vi "Practica 6 Alejandro Tejada ITIW31.vi"() -> ()   [LabVIEW 2018]
panel:
  in  "Eficiencia %":dbl
  out "Ganandia (dB)":dbl
  out "Longitud de onda":dbl
  in  "Frecuencia GHz (f)":dbl
  out "Area":dbl
  in  "Radio de la antena (r)":dbl
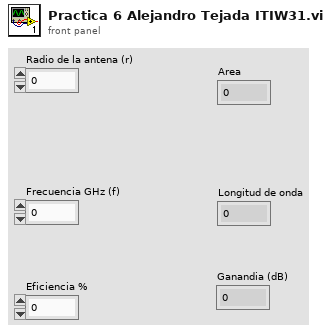
[diagram p1: front panel]
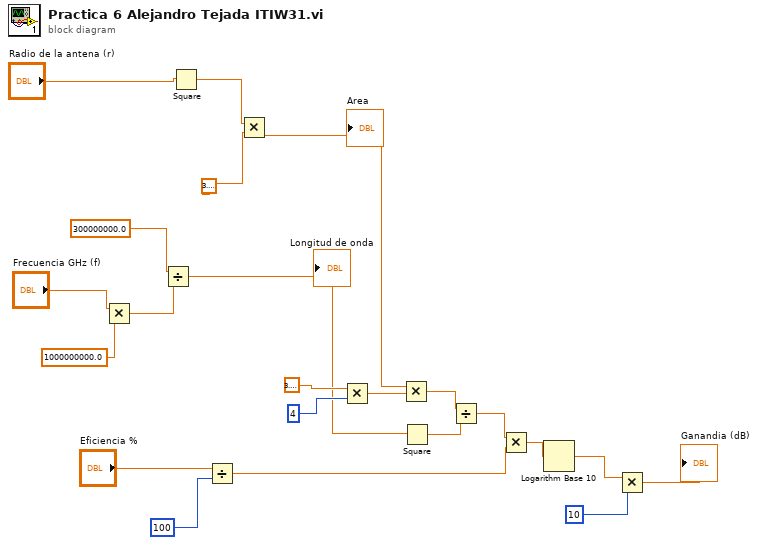
[diagram p0: block diagram]
diagram:
  n1 = Multiply(x="Frecuencia GHz (f)", y=1000000000.0) -> (x*y=w16:dbl)
  n2 = Divide(x=300000000.0, y=w16) -> (x/y=w9:dbl)
  "Longitud de onda" <- w9
  n3 = Square(x="Radio de la antena (r)") -> (x^2=w21:dbl)
  n4 = Divide(x="Eficiencia %", y=100) -> (x/y=w6:dbl)
  n5 = Multiply(x=w21, y=3.141592653589793) -> (x*y=w11:dbl)
  "Area" <- w11
  n6 = Multiply(x=3.141592653589793, y=4) -> (x*y=w10:dbl)
  n7 = Multiply(x=w11, y=w10) -> (x*y=w8:dbl)
  n8 = Square(x=w9) -> (x^2=w7:dbl)
  n9 = Divide(x=w8, y=w7) -> (x/y=w5:dbl)
  n10 = Multiply(x=w5, y=w6) -> (x*y=w2:dbl)
  n11 = Logarithm Base 10(1:w2) -> (0:w4:dbl)
  n12 = Multiply(x=w4, y=10) -> (x*y=→"Ganandia (dB)":dbl)
